vi "AlliGator Send Local Decay Plots (Parameter Map).vi"(8 "error in (no error)":errorcluster, 10 "ROI Descriptor":T1 {"Contours"."Type" items=["No Selection", "Point", "Line", "Rectangle", "Oval", "Polygon", "Freehand Region", "Annulus", "Unused2", "Unused3", "Broken Line", "Freehand Line", "Rotated Rectangle"]}, 11 "AlliGator IV DVR in":refnum<data-value>) -> (0 "error out":errorcluster, 3 "AlliGator IV DVR out":refnum<data-value>)   [LabVIEW 2021, in "AlliGator Local Decay Window.lvlib"]
doc: "Gets the data (decay, fit, IRF, residuals and fit parameters) at the selected ROI and sends it to the Local Decay Window for update."
uses:
  AlliGator Local Decay Window.lvlib
  Internal Variables/AlliGator Internal Variables v2.ctl
  <vilib>/vision/Image Controls.llb/IMAQ Image.ctl
  Internal Variables/AlliGator Gate Image Set.ctl
  Files/AlliGator FLI Dataset Type.ctl
  Files/AlliGator Data Series Type.ctl
  Dual-Channel Datasets/AlliGator Dataset Channel.ctl
  Settings/AlliGator Gate Arithmetic.ctl
  Source Image/AlliGator Displayed Image.ctl
  Image/Named ROI Description.ctl
  Phasor Graph/AlliGator Decay Metadata v3.ctl
  Decay Analysis/Decay Preprocessing/AlliGator Decay Background Subtraction Info.ctl
  Decay Analysis/Decay Preprocessing/AlliGator Baseline Subtraction Method.ctl
  Graphs/XY Graph/XY Graph Plot Shift Parameters.ctl
  Graphs/XY Graph/XY Graph Plot Shift Method.ctl
  Decay Analysis/Decay Preprocessing/AlliGator Decay Extrapolation Parameters.ctl
  Phasor/Calibration Phasor (m, phi).ctl
  Phasor/Phasor Reference Series.ctl
  Phasor/Phasor Calibration Map v2.ctl
  Phasor/Phasor (g, s).ctl
  Phasor Graph/AlliGator Raw Phasor Plot Data v5.ctl
  Phasor/Phasor Standard Deviation Options.ctl
  Phasor Plot/AlliGator Phasor Multi-Harmonic Data.ctl
  Phasor/Phasor Harmonic Data.ctl
  Decay Fit Parameter Map/AlliGator Decay Fit Options & Parameters v4.ctl
  Fits/IRF(X)PSED/Decay Fit Options v4.ctl
  Fits/Decay Convolution/Decay Model.ctl
  Fits/Residual Type.ctl
  Fits/IRF(X)PSED/Fit Weights Type v2.ctl
  Fits/Non-linear Fitting Method v2.ctl
  Fits/Fit Calculation Method.ctl
  Fits/Non-linear Fitting Algorithm.ctl
  Decay Analysis/Decay Fit/AlliGator Decay Fit Parameter Constraints 2.ctl
  Fits/IRF(X)PSED/Decay Fit Parameters In List.ctl
  Fits/IRF(X)PSED/MLE Baseline Offset Type.ctl
  Decay Analysis/Decay Preprocessing/AlliGator Decay Preprocessing Parameters.ctl
  Fits/IRF(X)PSED/Decay Fit Parameters & Derived Quantities List v2.ctl
  Fits/IRF(X)PSED/Decay Fit Result Constraint.ctl
  Decay Fit Parameter Map/AlliGator Parameter Maps Data.ctl
  Globals, Variables, Constants/AlliGator Globals, Variables & Constants.lvlib
  Globals, Variables, Constants/AlliGator Variables List.ctl
  Graphs/XY Graph/XY Graph Plot Data.ctl
  Graphs/XY Graph/XY Graph Add-Ons.lvlib
  Image Profile Window/AlliGator Image Profile Plot Data.ctl
  Image Profile Window/AlliGator Image Profile Window.lvlib
  Decay Analysis/Decay Processing/AlliGator Decay Processing.lvlib
  Time/Time.lvlib
  AlliGator Local Decay Fit Results.ctl
  AlliGator Local Decay Graph Window Event Refnum.ctl
  Decay Fit Parameter Map/AlliGator Decay Fit Parameter Map.lvlib
  Decay Analysis/Decay Preprocessing/AlliGator Decay Preprocessing.lvlib
  GUI/AlliGator GUI.lvlib
  Utilities/Read-Write.ctl
  Utilities/Utilities.lvlib
  Variant/Variant to Data/Variant to Data.lvlib
  Image/Image.lvlib
  Variant/Variant to Data/Variant to U16.vi
  Variant/Variant to Data/Variant to Boolean.vi
  Phasor/Phasor.lvlib
  Internal Variables/AlliGator Internal Variables.lvlib
  Files/AlliGator Files.lvlib
  Phasor Graph/AlliGator Phasor Graph.lvlib
  Phasor Plot/AlliGator Phasor Plot.lvlib
  Source Image/AlliGator Source Image.lvlib
  Fits/Fits.lvlib
  Decay Analysis/Decay Fit/AlliGator Decay Fit.lvlib
  Settings/AlliGator Settings.lvlib
  Dual-Channel Datasets/AlliGator Dual-Channel Datasets.lvlib
panel:
  out "CPU (s)":dbl
  # "see the AlliGator License on the block diagram (Ctrl+E or Window:Show Block Diagram)"
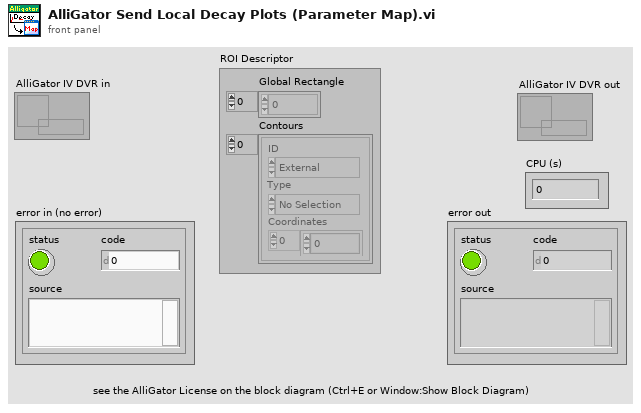
[diagram p1: front panel]
types:
  T1 = typedef "ROI Descriptor" = cluster{"Global Rectangle":i32[], "Contours":cluster{"ID":enum32{"External", "Internal"}, "Type":u32, "Coordinates":i32[]}[]}
  T2 = typedef "AlliGator Local Decay Window.lvlib/AlliGator Local Decay Graph Window Event Refnum.ctl" = refnum<user-event>
  T3 = typedef "AlliGator Globals, Variables & Constants.lvlib/AlliGator Variables List.ctl" = enum16{"---- GUI ----", "GUI:Initialization Status", "GUI:State Indicators Refnum", "GUI:Original AlliGator Menu Items", "GUI:Current Action Loop State", "GUI:Script in progress", "GUI:Playback", "GUI:Loop Playback", "GUI:Search ROI Used", "GUI:Search ROI", "Decay Graph Max Legend Size", "Intensity Graph Max Legend Size", "Decay Statistics Graph Max Legend Size", "Phasor Graph Max Legend Size", "Phasor Ratio Graph Max Legend Size", "Lifetime Graph Max Legend Size", "---- Files ----", "Files:Export Dataset Frames as Individual Files", "Files:Show Batch Export Help Balloons", "Files:Frames in Dataset", "Files:ptu File Frame Start Indices", "Files:Current Frame in Dataset", "Files:Current Frame Timestamp", "Files:Dataset Loaded", "Files:Dataset Metadata", "Files:Dataset Channel", "Files:Dataset Data Description", "Files:Background Dataset Metadata", "Files:Background Dataset Channel", "Files:Background Dataset Data Description", "Files:Background File Subtraction", "Files:Background File Path", "Files:Background File Pile-up Correction", "Files:Background File Pixel Well Capacity", "Files:Background File Scaling Factor", "Files:Current Dataset Load Settings", "Files:Dataset Path", "Files:ICCD-specific Information", "Files:Macrotime Gate Separation", "------ Python Plugins ------", "Python Plugins:Information", "Python Plugins:Python Session", "Python Plugins:Valid Python Session?", "---- Source Image ----", "Source Image:ROIs", "Source Image:Current ROI", "Source Image:ROI Event Refnum", "X_Source Image:Display Range", "X_Source Image:Palette Information", "X_Source Image:Type of Displayed Image", "X_Time Gate Slider", "Source Image:Palette List", "Source Image:Scale", "Source Image:ROI Overlay Color", "Source Image:Overlay to Erase", "Source Image:Is Displayed Image Accumulated", "Source Image:White Light Image Modified", "Source Image:Mask Image Modified", "---- Image Profile Window ----", "Image Profile:Window Event Refnum", "Image Profile:IntensityType", "Image Profile:Intensity Average Type", "Image Profile:Intensity-weighted SDV", "Image Profile:Box Profile Type", "Image Profile:Window Open", "Image Profile:Plotted Fit Parameter", "------ Phasor Graph -------", "Phasor Graph:Show Line", "---- Phasor Plot ---", "Phasor Plot:Parameters Changed", "Phasor Plot:FLI Dataset Modified since last Calculation", "Phasor Harmonics Data", "Selected Phasor Harmonics", "Phasor Harmonic Manager Event Refnum", "Phasor Plot:ROIs", "Phasor Plot:Current ROI", "Phasor Plot:ROI Event Refnum", "Phasor Plot:Image Reference Points", "Phasor Plot:Computed", "Phasor Plot:Palette Information", "Phasor Plot:Palette List", "Phasor Plot:Phasor Ratio Palette Information", "Phasor Plot:Phasor Ratio Palette List", "Phasor Plot:Image Scale", "Phasor Plot:Image Overlay to Erase", "Phasor Plot:Image Elements to Update", "Phasor Plot:Current Calculation Parameters", "Phasor Plot:Current Calibration Options", "Phasor Plot:Reset Cumulated Phasor Plot", "Phasor Plot:Reference 1", "Phasor Plot:Lifetime Reference 1", "Phasor Plot:Reference 1 Frequency", "Phasor Plot:Reference 2", "Phasor Plot:Lifetime Reference 2", "Phasor Plot:Reference 2 Frequency", "---- Decay Analysis ----", "Number of Selected Decays to Fit", "LS Fit Results", "LAR Fit Results", "BS Fit Results", "Last Decay Max - Min", "Best Fit Parameters", "Best Fit Parameter Names", "Actual Size X", "Actual Size Y", "Binning X", "Binning Y", "Actual # Gates", "Dataset Number", "Gates to...", "Gates Skipped", "Gates to keep", "Gate Step", "Gate Separation", "Reversed Gates", "Pile-up Correction", "Pixel Well Capacity", "Background Subtracted", "Background Subtraction Method", "Background Definition Range", "Background File (deprecated)", "Number of Dataset Accumulated", "Array of Accumulated Dataset Paths", "Do Averaged Datasets", "Destination File Path", "Process Plot Target", "Use 1/D as Phasor Frequency", "---- Decay Fit Parameter Map -----", "Decay Fit Parameter Map:Palette Information", "Decay Fit Parameter Map:Palette List", "Decay Fit Parameter Map:X Resolution", "Decay Fit Parameter Map:Y Resolution", "Decay Fit Parameter Map:Use Decay Fit Result Constraints", "Decay Fit Parameter Map:Decay Fit Result Constraints", "Decay Fit Parameter Map:Decay Fit Result Constraints Applied", "---- Parameter Map ----", "Parameter Map:Palette Information", "Parameter Map:Palette List", "------- Local Decay Window ---------", "Local Decay Graph Window:Event Refnum", "Local Decay Graph Window:Use normalized IRF for convolution", "----- Miscellaneous ----", "Misc:Skippable Dialog Windows Status"}
  T4 = typedef "IMAQ Image.ctl" = refnum<image>
  T5 = typedef "Utilities.lvlib/Read-Write.ctl" = enum16{"Read", "Write"}
  T6 = typedef "AlliGator Image Profile Window.lvlib/AlliGator Image Profile Plot Data.ctl" = cluster{"Plot Name":string, "Plot":T7}
  T7 = typedef "XY Graph Add-Ons.lvlib/XY Graph Plot Data.ctl" = cluster{"X Array":dbl[], "Y Array":dbl[]}
  T8 = typedef "AlliGator Internal Variables.lvlib/AlliGator Internal Variables v2.ctl" = cluster{"----------------------------- Images -----------------------------":u8, "Displayed Image":T4, "White Light Image":T4, "Mask Image":T4, "ROI Mask Image":T4, "Current Dataset Images 1":T9, "Background Dataset Images 1":T9, "Current Dataset Images 2":T9, "Background Dataset Images 2":T9, "Current Dataset Arithmetic Images":T9, "Accumulated Dataset Images 1":T9, "Accumulated Dataset Images 2":T9, "Accumulated Dataset Arithmetic Images":T9, "----------------------------- File Paths -----------------------------":u8, "Phasor Plot Image":T4, "Decay Fit Parameter Map Image":T4, "Parameter Map Image":T4, "Single Data Point Path":path, "White Light Image Path":path, "Mask Image Path":path, "Time-Series Folder":path, "[Time-Series Paths]":path[], "----------------------------- FLI Dataset -----------------------------":u8, "Current Dataset":i32, "Single Dataset Type":T10, "Current Folder":string, "AlliGator Data Series Type":T11, "# Datasets":i32, "Dual-Channel Dataset":bool, "Selected Channel Name":string, "Dataset Channel":T12, "Channel Arithmetic":T13, "Dual-Channel Background Dataset":bool, "Background Channel":T12, "Dual-Channel Accumulated Dataset":bool, "Start Time":dbl, "[Time-Series Timestamps]":dbl[], "[Intensity Corrections]":dbl[], "Time Series Script":bool, "Type of Displayed Image":T14, "Gate Image Slide":u16, "# Gates":i32, "ROIs":T15[], "----------------------------- Decays -----------------------------":u8, "ROI Decay":cluster{"t Array":dbl[], "I Array":dbl[]}, "Valid Decay":bool, "Decay  Metadata":T16, "Reference Decay Plot Name":string, "Reference Decay":cluster{"t Array":dbl[], "I Array":dbl[]}, "Decay Shift Plot":cluster{"Time Stamps":dbl[], "Decay Shifts":dbl[]}, "[Decays Max Values]":sgl[], "[Decays Min Values]":sgl[], "----------------------------- Calibration -----------------------------":u8, "Calibration Phasor":T22, "Calibration Phasor Series":T23, "Phasor Calibration Map":T24, "Calibration Map MD5 Digest":string, "----------------------------- Phasor Graph -----------------------------":u8, "Last Raw Phasor":T25, "Last Calibrated Phasor":T25, "Last Calibrated Phasor SDV":T25, "Phasor Graph:Phasor Plot":cluster{"g Array":dbl[], "s Array":dbl[]}, "Phasor Graph:Phasor SDV Plot":cluster{"g Array":dbl[], "s Array":dbl[]}, "[Phasor Graph:Raw Phasor Plots]":T26[], "Phasor Plot locked to Ref 1":i32, "[Phasor Plot(s) locked to Ref 1]":i32[], "[Phasor Plot(s) locked to Ref 2]":i32[], "[Pixel Phasors]":T25[], "----------------------------- Phasor Plot -----------------------------":u8, "[[Sum Image]]":dbl[][], "[[CSG Phasors]]":csg[][], "[[Valid Pixel?]]":bool[][], "[[Phasor Ratios]]":dbl[][], "[[Average Lifetimes]]":dbl[][], "Amplitude Weighted Average Lifetime":bool, "I/m/phi Dataset":cluster{"I/m/phi Dataset?":bool, "Base Frequency":dbl[unit], "Harmonic Orders":u8[]}, "Multi Phasor Plot Data":T28, "----------------------------- Decay Fit Parameter Map -----------------------------":u8, "Decay Fit Options & Parameters":T30, "Fit Options: Decay Preprocessing Parameters":T41, "Fit Options: Reference Decay":cluster{"t Array":dbl[], "I Array":dbl[]}, "Is Full Image Parameters Map":bool, "Is Single-Pixels Parameters Map":bool, "NLSF Parameters Map X Resolution":i32, "NLSF Parameters Map Y Resolution":i32, "[Single Decay Fit Parameters]":dbl[], "Fit Model":T32, "[[Multiple Decays Fit Parameters]]":dbl[][], "[[Multiple Decays Fit Parameter SDVs]]":dbl[][], "[[IRFs]]":dbl[][], "[ROI Descriptors]":T1[], "IRF Array Time Axis":dbl[], "Decay Array Time Axis":dbl[], "[Decay Fit Parameter Names]":T42[], "[Decay Sum]":dbl[], "Array of Decay Fit Result Constraints":T43[], "Selected ROIs Array":bool[], "----------------------------- Parameter Maps -----------------------------":u8, "[Map Set Names]":string[], "[Parameter Maps]":T44[], "[[User-defined Quantities]]":dbl[][], "User-defined Quantity":string}
  T9 = typedef "AlliGator Internal Variables.lvlib/AlliGator Gate Image Set.ctl" = cluster{"SGL Gate Images":T4[], "SGL Sum Image":T4, "SGL Max Image":T4, "SGL Min Image":T4}
  T10 = typedef "AlliGator Files.lvlib/AlliGator FLI Dataset Type.ctl" = enum16{"HDF5 FLI Dataset", "Gate Image Folder", ".sdt FLI Dataset (Becker & Hickl)", ".ptu FLI Dataset (PicoQuant)", "SS1 FLI Dataset", "SS2 FLI Dataset", "I/m/phi Dataset", ".bin FLI Dataset (PicoQuant Binned)", ".bin FLI Dataset (Piccolo Binned)", ".mat FLI Dataset"}
  T11 = typedef "AlliGator Files.lvlib/AlliGator Data Series Type.ctl" = enum16{"Not a Supported Series", "Gate Images Folder Series", "SwissSPAD 2 Dataset Series", "B&H FLI Dataset Series", "PicoQuant PTU FLI Dataset Series", "PicoQuant BIN FLI Dataset Series", "Piccolo hist BIN FLI Dataset Series", "HDF5 FLI Dataset Series"}
  T12 = typedef "AlliGator Dual-Channel Datasets.lvlib/AlliGator Dataset Channel.ctl" = enum16{"G2", "INT"}
  T13 = typedef "AlliGator Settings.lvlib/AlliGator Gate Arithmetic.ctl" = enum16{"None", "INT-G2", "G2/INT*<INT>", "(1 - G2/INT)*<INT>"}
  T14 = typedef "AlliGator Source Image.lvlib/AlliGator Displayed Image.ctl" = enum16{"Single Gate", "Sum of All Gates", "Max of All Gates", "Min of All Gates", "-", "White Ligth Image", "Mask Image"}
  T15 = typedef "Image.lvlib/Named ROI Description.ctl" = cluster{"ROI Descriptor":T1, "ROI Name":string, "Overlay Color":u32}
  T16 = typedef "AlliGator Phasor Graph.lvlib/AlliGator Decay Metadata v3.ctl" = cluster{"ROI Descriptor":T1, "ROI Center":cluster{"X":i32, "Y":i32}, "Decay Background Subtraction Info":T17, "Decay Reverted":bool, "Decay Smoothened":bool, "Decay Straightened":bool, "Fitted Tau (Decay Straightening)":dbl, "Decay Shift Parameters":T19, "Decay Shifted":bool, "Decay Extrapolated":bool, "Decay Extrapolation Parameters":T21, "Decay Normalized":bool, "Fold Decay":bool, "# Folds":u32}
  T17 = typedef "AlliGator Decay Preprocessing.lvlib/AlliGator Decay Background Subtraction Info.ctl" = cluster{"Laser Period":dbl[unit], "Gate Duration":dbl[unit], "Baseline Subtraction Method":T18, "Background Definition Range":cluster{"Min Gate":dbl[unit], "Max Gate":dbl[unit]}, "Total Intensity w/o Bkgd Subtraction":dbl, "Bkgd-subtracted Intensity (exp)":dbl, "# Data Points":i32, "Background/Gate":dbl, "Fitted Lifetime":dbl[unit], "Bkgd-subtracted Intensity (theo)":dbl}
  T18 = typedef "AlliGator Decay Preprocessing.lvlib/AlliGator Baseline Subtraction Method.ctl" = enum16{"Mean", "Min", "Square Gated Single-Exponential", "File", "Constant"}
  T19 = typedef "XY Graph Add-Ons.lvlib/XY Graph Plot Shift Parameters.ctl" = cluster{"Type":T20, "Shift":dbl[unit], "Threshold":dbl, "Rotate":bool}
  T20 = typedef "XY Graph Add-Ons.lvlib/XY Graph Plot Shift Method.ctl" = enum16{"Default", "CFD", "Threshold", "Cross-Correlation"}
  T21 = typedef "AlliGator Decay Preprocessing.lvlib/AlliGator Decay Extrapolation Parameters.ctl" = cluster{"Additional Points":u32, "Head Fraction":dbl, "Fitted Tau":dbl, "Use Periodicity":bool, "Use Cursors":bool, "Tail Fraction":dbl}
  T22 = typedef "Phasor.lvlib/Calibration Phasor (m, phi).ctl" = cluster{"m":dbl, "phi":dbl, "Phasor Frequency":dbl[unit], "Reference Lifetime":dbl[unit]}
  T23 = typedef "Phasor.lvlib/Phasor Reference Series.ctl" = cluster{"m Array":dbl[], "phi Array":dbl[], "Phasor Frequency":dbl[unit], "Calibration Lifetime":dbl[unit]}
  T24 = typedef "Phasor.lvlib/Phasor Calibration Map v2.ctl" = cluster{"Phasor Frequency":dbl[unit], "Calibration Lifetime":dbl[unit], "ROI Centers":cluster{"X":i32, "Y":i32}[], "ROI Descriptors":T1[], "Map Resolution X":i32, "Map Resolution Y":i32, "z Array":cdb[]}
  T25 = typedef "Phasor.lvlib/Phasor (g, s).ctl" = cluster{"g":dbl, "s":dbl}
  T26 = typedef "AlliGator Phasor Graph.lvlib/AlliGator Raw Phasor Plot Data v5.ctl" = cluster{"Phasor Plot Name":string, "Raw Phasor Plot":T25[], "Phasor Frequency":dbl[unit], "[Decay Metadata]":T16[], "Raw Phasor Plot SDV":T25[], "Phasor SDV Options":T27, "[Calibration Phasor]":T22[], "Intensity Array":dbl[]}
  T27 = typedef "Phasor.lvlib/Phasor Standard Deviation Options.ctl" = cluster{"Compute Estimated SDV":bool, "# Replicas":u32, "Use Estimated Average Phasor":bool}
  T28 = typedef "AlliGator Phasor Plot.lvlib/AlliGator Phasor Multi-Harmonic Data.ctl" = cluster{"Base Frequency":dbl[unit], "# Harmonics":u8, "Harmonic Orders":u8[], "Phasor Plot Settings Checksum":u64, "Phasor Harmonic Data Array":T29[]}
  T29 = typedef "Phasor.lvlib/Phasor Harmonic Data.ctl" = cluster{"Phasor Harmonic Name":string, "Phasor Plot Settings Checksum":u64, "Phasor Frequency":dbl[unit], "Base Frequency":dbl[unit], "Harmonic Order":u8, "Phasor Plot Parameters":string, "Phasor Array [[CSG]]":csg[][], "Dataset File Path":path}
  T30 = typedef "AlliGator Decay Fit Parameter Map.lvlib/AlliGator Decay Fit Options & Parameters v4.ctl" = cluster{"SYNC Period":dbl[unit], "Fit Options":T31, "Fit Parameter Constraints":T38[], "MLE Baseline Offset":dbl, "MLE Baseline Offset Type":T40}
  T31 = typedef "Fits.lvlib/Decay Fit Options v4.ctl" = cluster{"Show Fit Residuals":bool, "Fit Model":T32, "Residual Type":T33, "Max Decay Percentile":dbl, "Min Decay Percentile":dbl, "Show Full Decay":bool, "Weights":T34, "Fitting Method":T35, "Compute Parameter Uncertainties":bool, "Periodic Boundaries":bool, "Model Calculation":T36, "Period":dbl[unit], "Termination Criteria":cluster{"Max Iterations":i32, "Max Function Calls":i32, "Max Time":dbl[unit], "Function Tolerance":dbl, "Parameter Tolerance":dbl, "Gradient Tolerance":dbl, "Min Lambda":dbl, "Max Lambda":dbl, "Initial Tick Count":u32}, "Offset Resolution":dbl[unit], "Use Local IRF":bool, "Fitting Algorithm":T37, "Show Confidence Interval ":bool, "Confidence Level":dbl}
  T32 = typedef "Fits.lvlib/Decay Model.ctl" = enum16{"1-Exponential", "2-Exponentials"}
  T33 = typedef "Fits.lvlib/Residual Type.ctl" = enum16{"Standard", "Normalized", "Reduced"}
  T34 = typedef "Fits.lvlib/Fit Weights Type v2.ctl" = enum16{"Unweighted", "1/Variance (Neyman)", "1/Variance (Pearson)", "Best of All"}
  T35 = typedef "Fits.lvlib/Non-linear Fitting Method v2.ctl" = enum16{"Least Square", "Least Absolute Residual", "Bisquare", "MLE", "-", "Best of All"}
  T36 = typedef "Fits.lvlib/Fit Calculation Method.ctl" = enum16{"Simulation", "Convolution", "Integration"}
  T37 = typedef "Fits.lvlib/Non-linear Fitting Algorithm.ctl" = enum16{"Levenberg-Marquardt", "Trust-Region Dogleg"}
  T38 = typedef "AlliGator Decay Fit.lvlib/AlliGator Decay Fit Parameter Constraints 2.ctl" = cluster{"Fit Parameter":T39, "Min Value":dbl, "Max Value":dbl, "Global":bool, "Used":bool}
  T39 = typedef "Fits.lvlib/Decay Fit Parameters In List.ctl" = enum16{"Offset", "Baseline", "A_1", "tau_1", "A_2", "tau_2"}
  T40 = typedef "Fits.lvlib/MLE Baseline Offset Type.ctl" = enum32{"Absolute", "Percentage"}
  T41 = typedef "AlliGator Decay Preprocessing.lvlib/AlliGator Decay Preprocessing Parameters.ctl" = cluster{"Background Subtraction":bool, "Straighten Decay":bool, "Reverse Gates":bool, "1-Normalized Decay":bool, "Smoothen Decay":bool, "Smoothing Parameter":dbl, "Shift Decay":bool, "Decay Shift Parameters":T19, "Extrapolate Decay":bool, "Additional Points":u32, "Head Fraction":dbl, "Pixel-Normalize Decay":bool, "Use Periodicity":bool, "Use Cursors":bool, "Tail Fraction":dbl, "Use Decay Pre-Processing":bool, "Fold Decay":bool, "# Folds":u32, "[0-1]-Normalized Decay":bool}
  T42 = typedef "Fits.lvlib/Decay Fit Parameters & Derived Quantities List v2.ctl" = enum16{"Offset", "Baseline", "A_1", "tau_1", "A_2", "tau_2", "<tau>_a", "f1_a", "f2_a", "<tau>_i", "f1_i", "f2_i", "-", "R^2", "Chi^2"}
  T43 = typedef "Fits.lvlib/Decay Fit Result Constraint.ctl" = cluster{"Fit Parameter":enum16{"Offset", "Baseline", "A_1", "tau_1", "A_2", "tau_2", "<tau>_a", "f1_a", "f2_a", "<tau>_i", "f1_i", "f2_i", "-", "R^2", "Chi^2", "Max Relative Residual", "<Residual ACF>", "Residual ACF SDV", "tau_2/tau_1"}, "Min Value":dbl, "Max Value":dbl, "Use Constraint":bool}
  T44 = typedef "AlliGator Decay Fit Parameter Map.lvlib/AlliGator Parameter Maps Data.ctl" = cluster{"Map Set Name":string, "[Parameter Names]":string[], "[[Parameters]]":dbl[][], "[[Parameter SDVs]]":dbl[][], "Decay Array Time Axis":dbl[], "[[IRFs]]":dbl[][], "IRF Array Time Axis":dbl[], "X Resolution":i32, "Y Resolution":i32, "Intensity Array":dbl[]}
  T45 = cluster{"IRF Array Time Axis":dbl[], "[[IRFs]]":dbl[]}
  T46 = cluster{"t Axis":dbl[], "ROI Intensity Array":dbl[]}
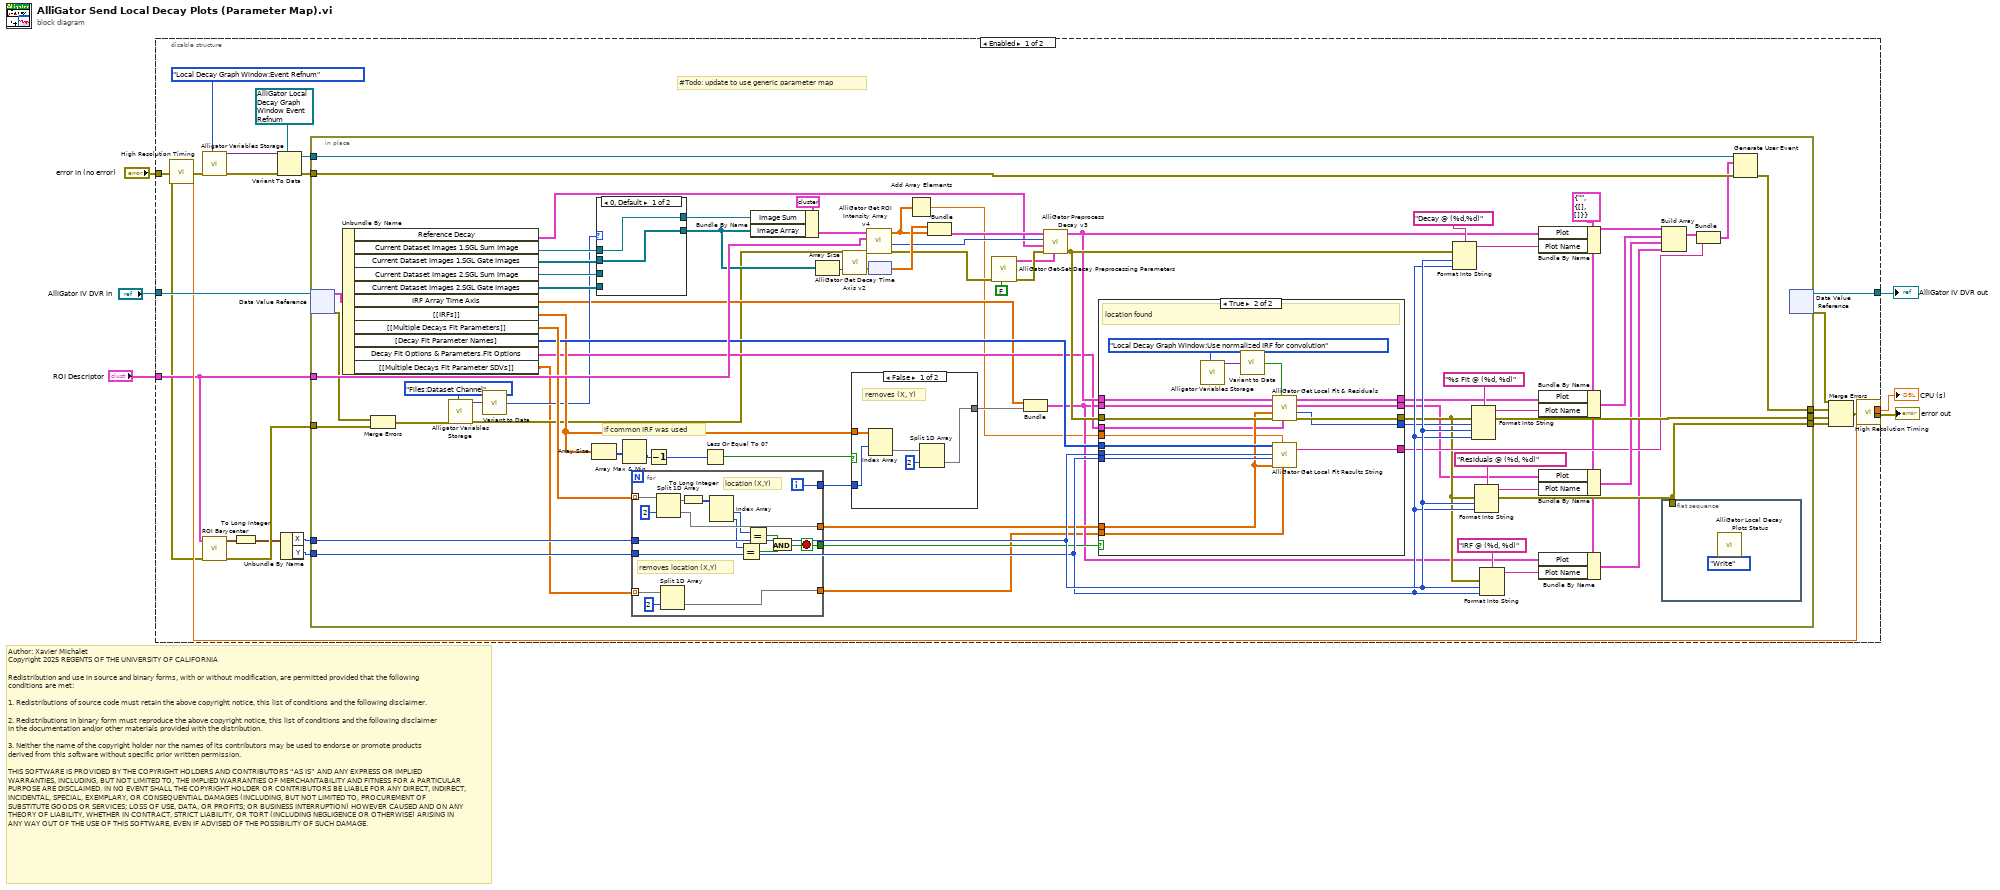
[diagram p0: block diagram]
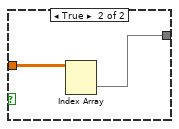
[diagram p3: hidden frame]
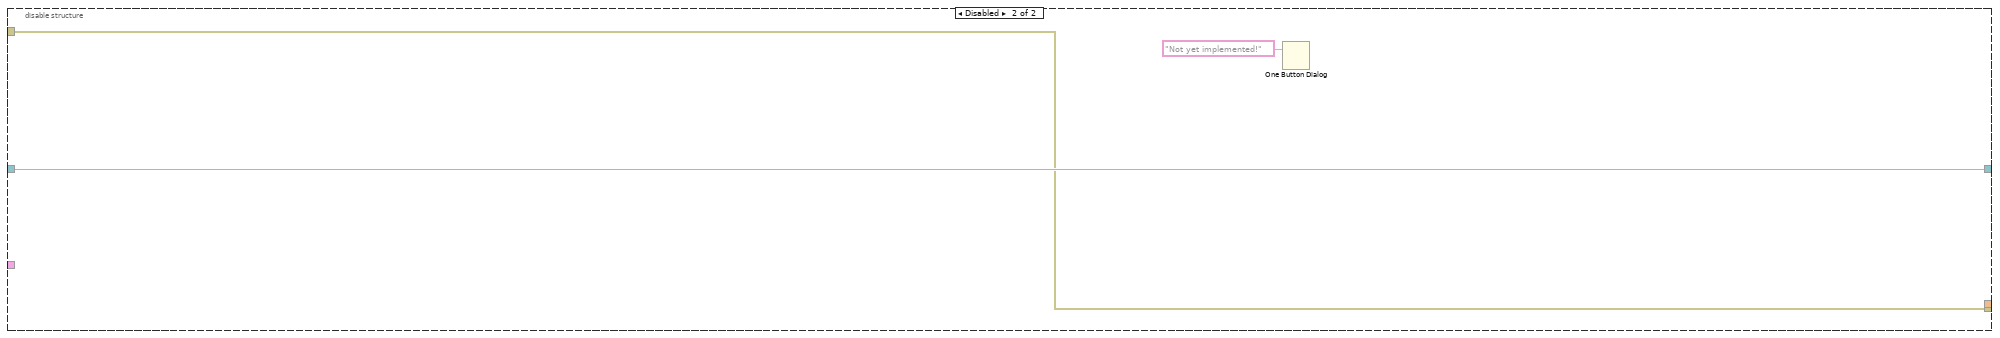
[diagram p5: hidden frame]
diagram:
  # "Author: Xavier Michalet\nCopyright 2025 REGENTS OF THE UNIVERSITY OF CALIFORNIA\n\nRedistribution and use in source and binary forms, with or without modification, are permitted provided that the following conditions are met:\n\n1. Redistributions of source code must retain the above copyright notice, this list of conditions and the following disclaimer.\n\n2. Redistributions in binary form must reproduce the above copyright notice, this list of conditions and the following disclaimer in the documentation and/or other materials provided with the distribution.\n\n3. Neither the name of the copyright holder nor the names of its contributors may be used to endorse or promote products derived from this software without specific prior written permission.\n\nTHIS SOFTWARE IS PROVIDED BY THE COPYRIGHT HOLDERS AND CONTRIBUTORS “AS IS” AND ANY EXPRESS OR IMPLIED WARRANTIES, INCLUDING, BUT NOT LIMITED TO, THE IMPLIED WARRANTIES OF MERCHANTABILITY AND FITNESS FOR A PARTICULAR PURPOSE ARE DISCLAIMED. IN NO EVENT SHALL THE COPYRIGHT HOLDER OR CONTRIBUTORS BE LIABLE FOR ANY DIRECT, INDIRECT, INCIDENTAL, SPECIAL, EXEMPLARY, OR CONSEQUENTIAL DAMAGES (INCLUDING, BUT NOT LIMITED TO, PROCUREMENT OF SUBSTITUTE GOODS OR SERVICES; LOSS OF USE, DATA, OR PROFITS; OR BUSINESS INTERRUPTION) HOWEVER CAUSED AND ON ANY THEORY OF LIABILITY, WHETHER IN CONTRACT, STRICT LIABILITY, OR TORT (INCLUDING NEGLIGENCE OR OTHERWISE) ARISING IN ANY WAY OUT OF THE USE OF THIS SOFTWARE, EVEN IF ADVISED OF THE POSSIBILITY OF SUCH DAMAGE."
  n1 = disable-structure shown="Enabled" {
    disable-tunnel: "AlliGator IV DVR in" -> [w30 w154]
    disable-tunnel: [w29 w154] -> w5
    disable-tunnel: [w17 w153] -> w4
    disable-tunnel: [w15 _] -> w3
    disable-tunnel: "ROI Descriptor" -> [w10 _]
    disable-tunnel: "error in (no error)" -> [w9 w153]
    frame Enabled {
      # "#Todo: update to use generic parameter map"
      n2 = call "High Resolution Timing.vi"("Error In"=w9) -> ("elapsed (relative) seconds"=w16:dbl, "Error Out"=w19:errorcluster)  [unwired: 16 in, 1 out]
      n3 = call "Alligator Variables Storage.vi"("AlliGator Variable"=AlliGator_Variables_List."Local Decay Graph Window:Event Refnum" ("Alligator Variable"), "Error In"=w19) -> ("Error Out"=w27:errorcluster, "Data out"=w25:variant)  [unwired: 7 in, 1 out]
      n4 = call "ROI Barycenter.vi"("Error In"=w9, "ROI Descriptor in"=w10) -> ("Error Out"=w8:errorcluster, "ROI Center"=w11:cluster{"X":dbl, "Y":dbl})  [unwired: 7 in, 1 out]
      n5 = To Long Integer(number=w11) -> (32bit integer=w7:cluster{"X":i32, "Y":i32})
      n6 = Variant To Data(error in=w27, type=T2 refnum ("Local Decay Graph Window Event Refnum"), Variant=w25) -> (data=w23:T2, error out=w26:errorcluster)
      n7 = Unbundle By Name(w7) -> ("X"=w21:i32, "Y"=w20:i32)
      n8 = in-place {
        in-place-border: w26 -> [w97]
        in-place-border: w23 -> [w103]
        in-place-border: [w102] -> w22
        in-place-border: w21 -> [w101]
        in-place-border: w20 -> [w100]
        in-place-border: w10 -> [w99]
        in-place-border: [w96] -> w14
        in-place-border: [w95] -> w13
        in-place-border: w8 -> [w94]
        w41 = T6 {"Plot Name"="", "Plot"={"X Array"=[], "Y Array"=[]}} ("Plot Data")
        # "if common IRF was used"
        n9 = in-place-dvr #1(w30) -> (w104:T8, w98:errorcluster)
        n10 = Unbundle By Name(w104) -> ("Reference Decay"=w35:cluster{"t Array":dbl[], "I Array":dbl[]}, "Current Dataset Images 1.SGL Sum Image"=w57:T4, "Current Dataset Images 1.SGL Gate Images"=w60:T4[], "Current Dataset Images 2.SGL Sum Image"=w56:T4, "Current Dataset Images 2.SGL Gate Images"=w59:T4[], "IRF Array Time Axis"=w43:dbl[], "[[IRFs]]"=w50:dbl[][], "[[Multiple Decays Fit Parameters]]"=w78:dbl[][], "[Decay Fit Parameter Names]"=w75:T42[], "Decay Fit Options & Parameters.Fit Options"=w47:T31, "[[Multiple Decays Fit Parameter SDVs]]"=w32:dbl[][])
        n11 = Merge Errors(w98, w94) -> (w36:errorcluster)
        n12 = call "Alligator Variables Storage.vi"("AlliGator Variable"=AlliGator_Variables_List."Files:Dataset Channel" ("Alligator Variable"), "Error In"=w36) -> ("Error Out"=w37:errorcluster, "Data out"=w45:variant)  [unwired: 7 in, 1 out]
        n13 = call-poly "Variant to Data.vi"("Variant"=w45) -> ("U16 Value"=w44:u16)  [unwired: 8 in]
        n14 = Array Size(array=w50) -> (size(s)=w54:i32[])
        n15 = case shown="0, Default" w44 {
          tunnel: [w107 w109] -> w55
          tunnel: w56 -> [_ w109]
          tunnel: w59 -> [_ w108]
          tunnel: [w106 w108] -> w58
          tunnel: w57 -> [w107 _]
          tunnel: w60 -> [w106 _]
          frame 0, Default {
          }
          frame 1 {
          }
        }
        n16 = Array Max & Min(array=w54) -> (min value=w53:i32)  [unwired: 3 out]
        n17 = for {
          tunnel: w78 -> [w151] mode=indexing
          tunnel: w101 -> [w150]
          tunnel: w100 -> [w149]
          tunnel: [w148] -> w84
          tunnel: [w147] -> w79
          tunnel: [w141] -> w49
          tunnel: w32 -> [w137] mode=indexing
          tunnel: [w136] -> w31
          i -> [w141]
          stop <- w148 stop-if-true
          # "location (X,Y)"
          # "removes location (X,Y)"
          n18 = Split 1D Array(array=w151, index=2) -> (first subarray=w140:dbl[], second subarray=w147:dbl[])
          n19 = Split 1D Array(array=w137, index=2) -> (second subarray=w136:dbl[])  [unwired: 1 out]
          n20 = To Long Integer(number=w140) -> (32bit integer=w139:i32[])
          n21 = Index Array(array=w139) -> (element #1=w145:i32, element #2=w144:i32)  [unwired: 2 in]
          n22 = Equal?(x=w144, y=w149) -> (x = y?=w142:bool)
          n23 = Equal?(x=w145, y=w150) -> (x = y?=w143:bool)
          n24 = And(x=w143, y=w142) -> (x .and. y?=w148:bool)
        }
        n25 = Decrement(x=w53) -> (x-1=w52:i32)
        n26 = Less Or Equal To 0?(x=w52) -> (x <= 0?=w51:bool)
        n27 = Bundle By Name(cluster=cluster{"Image Sum":T4, "Image Array":T4[]} {"Image Sum"=refnum, "Image Array"=[]} ("Images"), "Image Sum"=w55, "Image Array"=w58) -> (w82:cluster{"Image Sum":T4, "Image Array":T4[]})
        n28 = Array Size(array=w58) -> (size(s)=w81:i32)
        n29 = call "AlliGator Get Decay Time Axis v2.vi"("Number of Gates"=w81) -> ("t Array"=w80:dbl[unit][])  [unwired: 14 in]
        n30 = case shown="False" w51 {
          tunnel: w50 -> [w114 w116]
          tunnel: [w111 w115] -> w42
          tunnel: w49 -> [w113 _]
          frame False {
            # "removes (X, Y)"
            n31 = Index Array(array=w114, index (row)=w113) -> (element=w112:dbl[])  [unwired: 1 in]
            n32 = Split 1D Array(array=w112, index=2) -> (second subarray=w111:dbl[])  [unwired: 1 out]
          }
          frame True {
            n33 = Index Array(array=w116) -> (element=w115:dbl[])  [unwired: 2 in]
          }
        }
        n34 = call "AlliGator Get ROI Intensity Array v4.vi"("error in (no error)"=w37, "ROI Descriptor"=w99, "Images"=w82) -> ("Error Out"=w68:errorcluster, "# Valid Pixels"=w66:i32, "ROI Intensity Array"=w34:dbl[])  [unwired: 3 in, 3 out]
        n35 = node(w80) -> (w77:dbl[])
        n36 = Add Array Elements(numeric array=w34) -> (sum=w33:dbl)
        n37 = Bundle(w77, "ROI Intensity Array"=w34) -> (w65:cluster{dbl[], "ROI Intensity Array":dbl[]})  [unwired: 1 in]
        n38 = call "AlliGator Get-Set Decay Preprocessing Parameters.vi"("Get (F)/Set"=FALSE, "Error In"=w68) -> ("Error Out"=w67:errorcluster, "Decay Preprocessing Parameters out"=w63:T41)  [unwired: 8 in]
        n39 = Bundle("IRF Array Time Axis"=w43, "[[IRFs]]"=w42) -> (w38:T45)  [unwired: 1 in]
        n40 = call "AlliGator Preprocess Decay v3.vi"("Decay Preprocessing Parameters"=w63, "Error In"=w67, "Time-Gated Reference Decay"=w35, "# Pixels"=w66, "Decay (in)"=w65) -> ("Error Out"=w64:errorcluster, "Decay (out)"=w61:T46)  [unwired: 3 in, 2 out]
        n41 = case shown="True" w84 {
          tunnel: w79 -> [_ w127]
          tunnel: w64 -> [w117 w135]
          tunnel: [w117 w134] -> w48
          tunnel: w61 -> [_ w133]
          tunnel: [_ w132] -> w76
          tunnel: w75 -> [_ w131]
          tunnel: w101 -> [_ w130]
          tunnel: w100 -> [_ w129]
          tunnel: [_ w128] -> w73
          tunnel: w47 -> [_ w126]
          tunnel: w38 -> [_ w125]
          tunnel: [_ w124] -> w40
          tunnel: [_ w123] -> w39
          tunnel: w33 -> [_ w119]
          tunnel: w31 -> [_ w118]
          frame False {
            # "Not a valid location"
          }
          frame True {
            # "location found"
            n42 = call "Alligator Variables Storage.vi"("AlliGator Variable"=AlliGator_Variables_List."Local Decay Graph Window:Use normalized IRF for convolution") -> ("Data out"=w122:variant)  [unwired: 8 in, 2 out]
            n43 = call-poly "Variant to Data.vi"("Variant"=w122) -> ("Value"=w120:bool)  [unwired: 8 in]
            n44 = call "AlliGator Get Local Fit & Residuals.vi"("Fit Options"=w126, "Use Normalized IRF (T)"=w120, "Error In"=w135, "All Fit Parameters (w tau)"=w127, "IRF"=w125, "Decay Plot"=w133) -> ("Error Out"=w134:errorcluster, "Fit Model"=w132:T32, "Residual Plot"=w123:cluster{"X Array":dbl[], "Y Array":dbl[]}, "Fit Plot"=w124:cluster{"X Array":dbl[], "Y Array":dbl[]})  [unwired: 2 in]
            n45 = call "AlliGator Get Local Fit Results String.vi"("Parameters SDV"=w118, "Decay Sum"=w119, "Parameters"=w127, "Y"=w129, "X"=w130, "[Decay Fit Parameter Name]"=w131) -> ("Fit Results String"=w128:string)  [unwired: 5 in]
          }
        }
        n46 = Format Into String(format string="Decay @ (%d,%d)" ("Plot Name"), error in=w64, w101, w100) -> (resulting string=w90:string)  [unwired: 1 in, 1 out]
        n47 = Format Into String(format string="%s Fit @ (%d, %d)" ("Plot Name"), error in=w48, w76, w101, w100) -> (resulting string=w87:string, error out=w96:errorcluster)  [unwired: 1 in]
        n48 = Format Into String(format string="Residuals @ (%d, %d)" ("Plot Name"), error in=w48, w101, w100) -> (resulting string=w85:string, error out=w95:errorcluster)  [unwired: 1 in]
        n49 = Format Into String(format string="IRF @ (%d, %d)" ("Plot Name"), error in=w48, w101, w100) -> (resulting string=w70:string)  [unwired: 1 in, 1 out]
        n50 = Bundle By Name(cluster=w41, "Plot"=w61, "Plot Name"=w90) -> (w93:T6)
        n51 = Bundle By Name(cluster=w41, "Plot"=w40, "Plot Name"=w87) -> (w92:T6)
        n52 = Bundle By Name(cluster=w41, "Plot"=w39, "Plot Name"=w85) -> (w91:T6)
        n53 = Bundle By Name(cluster=w41, "Plot"=w38, "Plot Name"=w70) -> (w69:T6)
        n54 = Build Array(w93, w92, w91, w69) -> (w74:T6[])
        n55 = flat-sequence {
          tunnel: w95 -> [_]
          frame #0 {
            n56 = call "AlliGator Local Decay Plots Status.vi"("Read/Write"=Read-Write."Write") -> ()  [unwired: 8 in, 1 out]
          }
        }
        n57 = Bundle(w74, "Fit Results String"=w73) -> (w72:cluster{T6[], "Fit Results String":string})  [unwired: 1 in]
        n58 = Generate User Event(user event=w103, event data cluster=w72, error in=w97) -> (error out=w102:errorcluster)  [unwired: 1 in, 1 out]
        n59 = in-place-dvr #1() -> (w29:refnum<data-value>, w12:errorcluster)  [unwired: 1 in]
      }
      n60 = Merge Errors(w12, w22, w14, w13) -> (w18:errorcluster)
      n61 = call "High Resolution Timing.vi"("relative seconds (NaN)"=w16, "Error In"=w18) -> ("elapsed (relative) seconds"=w15:dbl, "Error Out"=w17:errorcluster)  [unwired: 15 in, 1 out]
    }
    frame Disabled {
      n62 = One Button Dialog(message="Not yet implemented!") -> ()  [unwired: 1 in, 1 out]
    }
  }
  "error out" <- w4
  "AlliGator IV DVR out" <- w5
  "CPU (s)" <- w3
